vi "IPS120_CloseHeater.vi"(0 "Instrument address (in)":T1={"Com Port"=1, "ISOBUS Address"=1, "GPIB Address"=24, "Communication"=enum."ISOBUS"}, 1 "Last run?":bool, 2 "B field Change?":bool, 3 "error in":errorcluster, 4 "Hold(min)":dbl) -> (5 "error out":errorcluster)   [LabVIEW 2012]
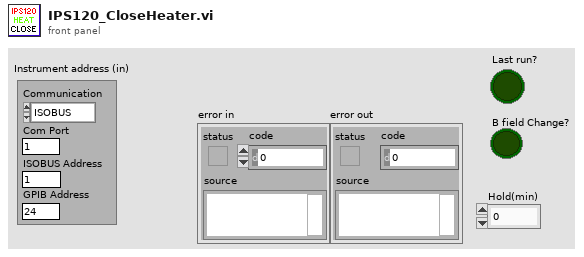
[diagram p1: front panel]
types:
  T1 = cluster{"Com Port":i32, "ISOBUS Address":i32, "GPIB Address":i16, "Communication":enum16{"RS232", "ISOBUS", "GPIB", "Gateway"}}
  T2 = typedef "OxfordAddress.ctl" = cluster{"Com Port":i32, "ISOBUS Address":i32, "GPIB Address":i16, "Communication":enum16{"RS232", "ISOBUS", "GPIB", "Gateway"}}
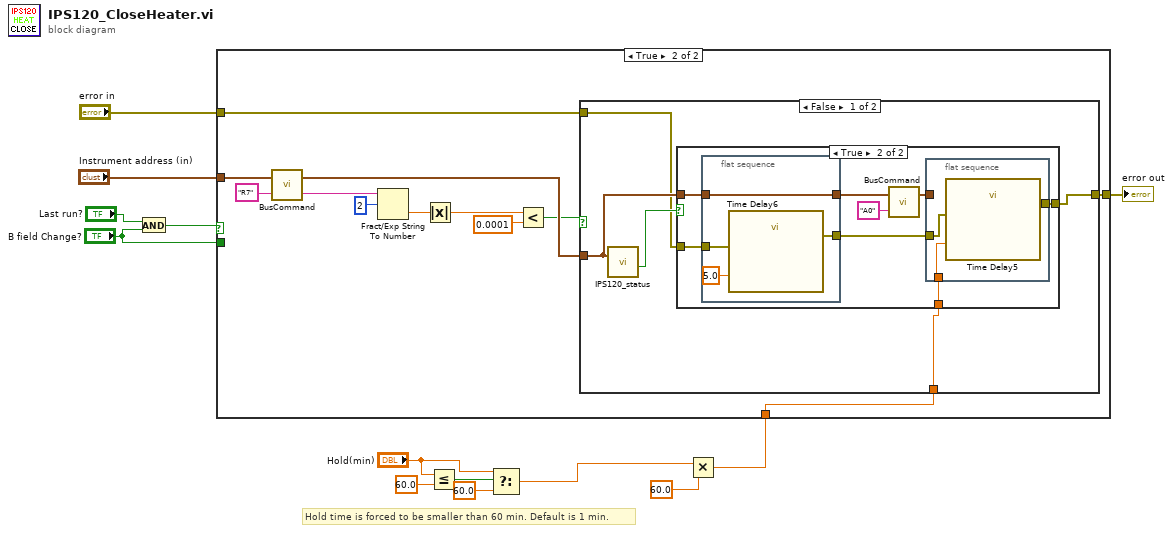
[diagram p0: block diagram]
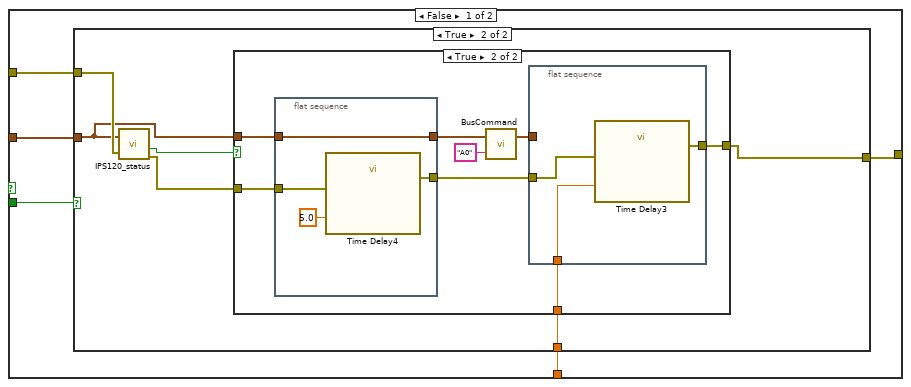
[diagram p2: hidden frame]
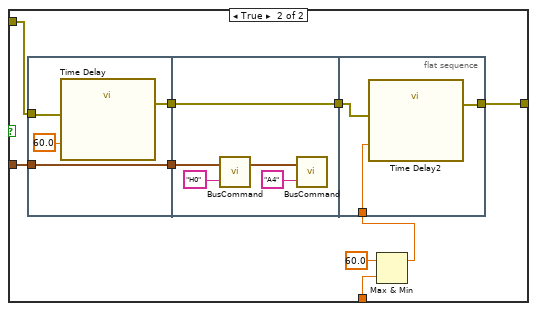
[diagram p6: hidden frame]
diagram:
  # "Hold time is forced to be smaller than 60 min. Default is 1 min."
  n1 = And(x="Last run?", y="B field Change?") -> (x .and. y?=w11:bool)
  n2 = Less Or Equal?(x="Hold(min)", y=60.0) -> (x <= y?=w5:bool)
  n3 = Select(t="Hold(min)", s=w5, f=60.0) -> (s? t:f=w3:dbl)
  n4 = Multiply(x=w3, y=60.0) -> (x*y=w7:dbl)
  n5 = case shown="True" w11 {
    tunnel: "Instrument address (in)" -> [w17 w45]
    tunnel: [w15 w44] -> w12
    tunnel: "error in" -> [w16 w43]
    tunnel: "B field Change?" -> [w18 _]
    tunnel: w7 -> [w14 w42]
    frame False {
      n6 = case shown="True" w18 {
        tunnel: w17 -> [_ w23]
        tunnel: w16 -> [w19 w25]
        tunnel: [w19 w21] -> w15
        tunnel: w14 -> [_ w20]
        frame False {
        }
        frame True {
          n7 = call "IPS120_status.vi"("Address"=w23, "error in"=w25) -> ("Arrive"=w24:bool, "error out"=w22:errorcluster)  [unwired: 4 out]
          n8 = case shown="True" w24 {
            tunnel: w23 -> [_ w32]
            tunnel: w22 -> [w26 w30]
            tunnel: [w26 w28] -> w21
            tunnel: w20 -> [_ w27]
            frame False {
            }
            frame True {
              n9 = flat-sequence {
                tunnel: w32 -> [w37]
                tunnel: [w37] -> w31
                tunnel: w30 -> [w36]
                tunnel: [w35] -> w29
                frame #0 {
                  n10 = call "Time Delay4"("error in (no error)"=w36, "Delay Time (s)"=5.0) -> ("error out"=w35:errorcluster)  [unwired: 9 in]
                }
              }
              n11 = call "BusCommand.vi"("Command"="A0", "Instrument address (in)"=w31) -> ("Instrument address (out)"=w33:T2)  [unwired: 1 out]
              n12 = flat-sequence {
                tunnel: w33 -> [_]
                tunnel: w29 -> [w41]
                tunnel: [w40] -> w28
                tunnel: w27 -> [w39]
                frame #0 {
                  n13 = call "Time Delay3"("error in (no error)"=w41, "Delay Time (s)"=w39) -> ("error out"=w40:errorcluster)  [unwired: 9 in]
                }
              }
            }
          }
        }
      }
    }
    frame True {
      n14 = call "BusCommand.vi"("Command"="R7", "Instrument address (in)"=w45) -> ("Reply"=w52:string, "Instrument address (out)"=w47:T2)
      n15 = Fract/Exp String To Number(string=w52, offset=2) -> (number=w49:dbl)  [unwired: 2 in, 1 out]
      n16 = Absolute Value(x=w49) -> (abs(x)=w50:dbl)
      n17 = Less?(x=w50, y=0.0001) -> (x < y?=w46:bool)
      n18 = case shown="False" w46 {
        tunnel: w47 -> [w57 w81]
        tunnel: [w55 w80] -> w44
        tunnel: w43 -> [w56 w79]
        tunnel: w42 -> [w54 w77]
        frame False {
          n19 = call "IPS120_status.vi"("Address"=w57) -> ("Arrive"=w58:bool)  [unwired: 1 in, 5 out]
          n20 = case shown="True" w58 {
            tunnel: w57 -> [_ w65]
            tunnel: w56 -> [w59 w63]
            tunnel: [w59 w61] -> w55
            tunnel: w54 -> [_ w60]
            frame False {
            }
            frame True {
              n21 = flat-sequence {
                tunnel: w65 -> [w70]
                tunnel: [w70] -> w64
                tunnel: w63 -> [w69]
                tunnel: [w68] -> w62
                frame #0 {
                  n22 = call "Time Delay6"("error in (no error)"=w69, "Delay Time (s)"=5.0) -> ("error out"=w68:errorcluster)  [unwired: 9 in]
                }
              }
              n23 = call "BusCommand.vi"("Command"="A0", "Instrument address (in)"=w64) -> ("Instrument address (out)"=w66:T2)  [unwired: 1 out]
              n24 = flat-sequence {
                tunnel: w66 -> [_]
                tunnel: w62 -> [w74]
                tunnel: [w73] -> w61
                tunnel: w60 -> [w72]
                frame #0 {
                  n25 = call "Time Delay5"("error in (no error)"=w74, "Delay Time (s)"=w72) -> ("error out"=w73:errorcluster)  [unwired: 9 in]
                }
              }
            }
          }
        }
        frame True {
          n26 = flat-sequence {
            tunnel: w81 -> [w87]
            tunnel: [w87] -> w83
            tunnel: w79 -> [w85]
            tunnel: [w84] -> w82
            tunnel: w83 -> [w89]
            tunnel: w82 -> [w88]
            tunnel: [w88] -> w78
            tunnel: [w94] -> w80
            tunnel: w78 -> [w95]
            tunnel: w75 -> [w93]
            frame #0 {
              n27 = call "Time Delay"("error in (no error)"=w85, "Delay Time (s)"=60.0) -> ("error out"=w84:errorcluster)  [unwired: 9 in]
            }
            frame #1 {
              n28 = call "BusCommand.vi"("Command"="H0", "Instrument address (in)"=w89) -> ("Instrument address (out)"=w91:T2)  [unwired: 1 out]
              n29 = call "BusCommand.vi"("Command"="A4", "Instrument address (in)"=w91) -> ()  [unwired: 2 out]
            }
            frame #2 {
              n30 = call "Time Delay2"("error in (no error)"=w95, "Delay Time (s)"=w93) -> ("error out"=w94:errorcluster)  [unwired: 9 in]
            }
          }
          n31 = Max & Min(x=60.0, y=w77) -> (max(x,y)=w75:dbl)  [unwired: 1 out]
        }
      }
    }
  }
  "error out" <- w12
